vi "Include Default Region in URL.vi"(11 "Bucket":refnum<class "Bucket.lvclass">) -> (3 "Include Default Region":bool)   [LabVIEW 2015, in "NI_AWS_S3.lvlib" / "Bucket.lvclass"]
uses:
  Bucket.lvclass
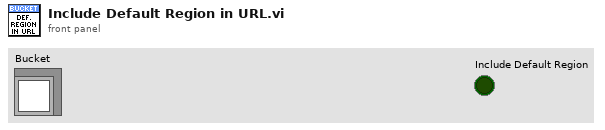
[diagram p1: front panel]
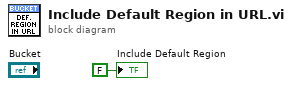
[diagram p0: block diagram]
diagram:
  "Include Default Region" <- FALSE ("Include Default Region")
